vi "dfd_FXPSimu Casting (vector).vi"(7 "FXP op":T4={"source"=6, "is floating?"=FALSE, "o-mode"=enum."Wrap", "q-mode"=enum."Nearest", "signed?"=FALSE, "fwl"=0, "high limit"=0.0, "low limit"=0.0, "full range"=0.0} {"source" items=["Coef a/k"=0, "Coef b/v"=7, "Input"=1, "Output"=2, "Multiplicand"=3, "Product"=4, "Sum"=5, "Delay"=6, "Gain"=8]}, 8 "filtering statistics in":T3(array[cluster]) {"statistics information"."min value" format="%.2f"; "statistics information"."max value" format="%.2f"; "Quantizer Source" items=["Coefficients a/k"=0, "Coefficients b/v"=7, "Input"=1, "Output"=2, "Multiplicand"=3, "Product"=4, "Sum"=5, "Delay"=6]}, 11 "values in":ext[](array[numeric]) format="%.2f") -> (0 "filtering statistics out":T3(array[cluster]) {"statistics information"."min value" format="%.2f"; "statistics information"."max value" format="%.2f"; "Quantizer Source" items=["Coefficients a/k"=0, "Coefficients b/v"=7, "Input"=1, "Output"=2, "Multiplicand"=3, "Product"=4, "Sum"=5, "Delay"=6]}, 3 "values out":ext[](array[numeric]) format="%.2f")   [LabVIEW 2017, in "NI_DigFilter_FXP.lvlib"]
uses:
  <vilib>/addons/Digital Filter Design/NI_DigFilter_FXP.lvlib
  <vilib>/addons/Digital Filter Design/_Objects.llb/dfd_FXP Operation.ctl
  <vilib>/addons/Digital Filter Design/_Objects.llb/dfd_Internal Quantization Srcs.ctl
  <vilib>/addons/Digital Filter Design/_Objects.llb/DFD Quantization Sources.ctl
  <vilib>/addons/Digital Filter Design/_Objects.llb/DFD FXP Statistics Data.ctl
  <vilib>/addons/Digital Filter Design/NI_DigFilterLicensed.lvlib
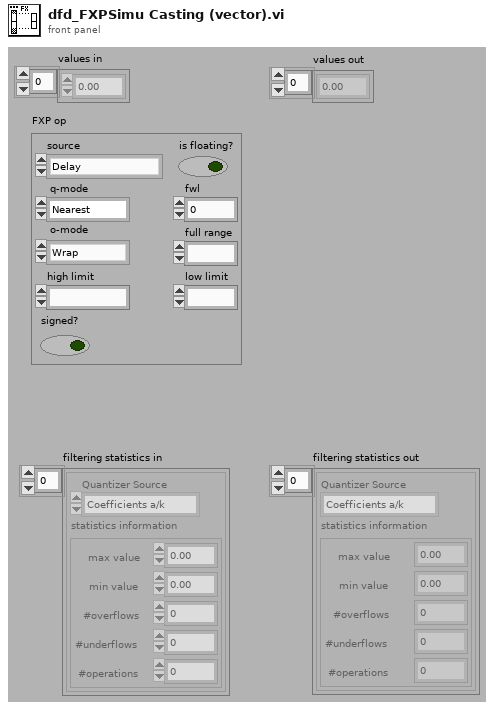
[diagram p1: front panel]
types:
  T1 = typedef "NI_DigFilterLicensed.lvlib/DFD Quantization Sources.ctl" = u16
  T2 = typedef "NI_DigFilterLicensed.lvlib/DFD FXP Statistics Data.ctl" = cluster{"max value":ext, "min value":ext, "#overflows":i32, "#underflows":i32, "#operations":i32}
  T3 = cluster{"Quantizer Source":T1, "statistics information":T2}[]
  T4 = typedef "dfd_FXP Operation.ctl" = cluster{"source":T5, "is floating?":bool, "o-mode":enum16{"Saturation", "Wrap"}, "q-mode":enum16{"Nearest", "Truncation"}, "signed?":bool, "fwl":i16, "high limit":ext, "low limit":ext, "full range":ext}
  T5 = typedef "NI_DigFilterLicensed.lvlib/dfd_Internal Quantization Srcs.ctl" = u16
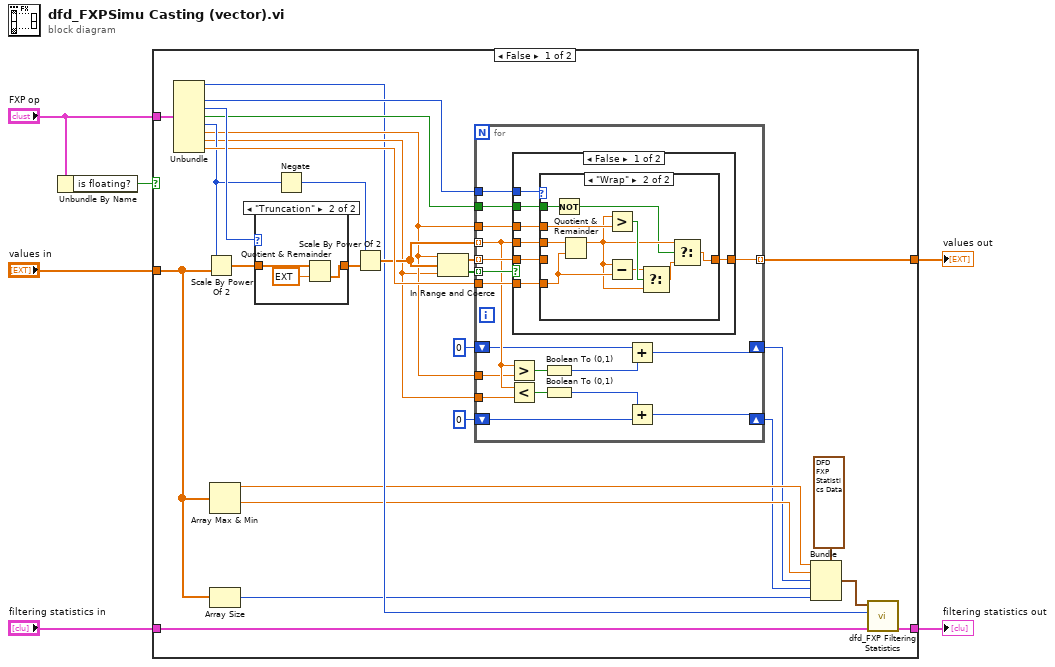
[diagram p0: block diagram]
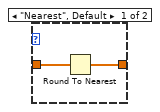
[diagram p4: hidden frame]
diagram:
  n1 = Unbundle By Name("FXP op") -> ("is floating?"=w1:bool)
  n2 = case shown="False" w1 {
    tunnel: [w34 w78] -> w6
    tunnel: "FXP op" -> [w33 _]
    tunnel: "filtering statistics in" -> [w8 w77]
    tunnel: "values in" -> [w24 w78]
    tunnel: [w7 w77] -> w2
    frame False {
      n3 = Unbundle(w33) -> ("source"=w16:T5, "o-mode"=w26:enum16{"Saturation", "Wrap"}, "q-mode"=w31:enum16{"Nearest", "Truncation"}, "signed?"=w27:bool, "fwl"=w22:i16, "high limit"=w20:ext, "low limit"=w19:ext, "full range"=w28:ext)  [unwired: 1 out]
      n4 = Scale By Power Of 2(n=w22, x=w24) -> (x*2^n=w32:ext[])
      n5 = Array Max & Min(array=w24) -> (max value=w14:ext, min value=w13:ext)  [unwired: 2 out]
      n6 = Array Size(array=w24) -> (size(s)=w10:i32)
      n7 = case shown="\"Truncation\"" w31 {
        tunnel: w32 -> [w73 w76]
        tunnel: [w72 w74] -> w25
        frame "Nearest", Default {
          n8 = Round To Nearest(number=w73) -> (nearest integer value=w72:ext[])
        }
        frame "Truncation" {
          n9 = Quotient & Remainder(x=w76, y=ext 1.0) -> (floor(x/y)=w74:ext[])  [unwired: 1 out]
        }
      }
      n10 = Negate(x=w22) -> (-x=w21:i16)
      n11 = Scale By Power Of 2(n=w21, x=w25) -> (x*2^n=w23:ext[])
      n12 = In Range and Coerce(upper limit=w20, x=w23, lower limit=w19) -> (coerced(x)=w29:ext[], In Range?=w30:bool[])
      n13 = for {
        tunnel: [w52] -> w34 mode=indexing
        tunnel: w30 -> [w51] mode=indexing
        tunnel: w29 -> [w50] mode=indexing
        tunnel: w20 -> [w49]
        tunnel: w28 -> [w48]
        tunnel: w27 -> [w47]
        tunnel: w26 -> [w46]
        tunnel: w23 -> [w45] mode=indexing
        tunnel: w20 -> [w44]
        tunnel: w19 -> [w43]
        shift-right: [w36] -> w12
        shift-left: 0 -> [w40]
        shift-right: [w35] -> w11
        shift-left: 0 -> [w38]
        n14 = Greater?(x=w45, y=w44) -> (0:w42:bool)
        n15 = Less?(x=w45, y=w43) -> (x < y?=w41:bool)
        n16 = case shown="False" w51 {
          tunnel: [w57 w71] -> w52
          tunnel: w50 -> [w58 w71]
          tunnel: w46 -> [w59 _]
          tunnel: w48 -> [w56 _]
          tunnel: w45 -> [w55 _]
          tunnel: w47 -> [w54 _]
          tunnel: w49 -> [w53 _]
          frame False {
            n17 = case shown="\"Wrap\"" w59 {
              tunnel: [w60 w69] -> w57
              tunnel: w58 -> [w60 _]
              tunnel: w56 -> [_ w64]
              tunnel: w55 -> [_ w70]
              tunnel: w54 -> [_ w68]
              tunnel: w53 -> [_ w67]
              frame "Saturation", Default {
              }
              frame "Wrap" {
                n18 = Not(x=w68) -> (.not. x?=w61:bool)
                n19 = Quotient & Remainder(x=w70, y=w64) -> (x-y*floor(x/y)=w63:ext)  [unwired: 1 out]
                n20 = Greater?(x=w63, y=w67) -> (0:w66:bool)
                n21 = Subtract(x=w63, y=w64) -> (x-y=w65:ext)
                n22 = Select(t=w65, s=w66, f=w63) -> (s? t:f=w62:ext)
                n23 = Select(t=w63, s=w61, f=w62) -> (s? t:f=w69:ext)
              }
            }
          }
          frame True {
          }
        }
        n24 = Boolean To (0,1)(Boolean=w42) -> (0, 1=w39:i16)
        n25 = Boolean To (0,1)(Boolean=w41) -> (0, 1=w37:i16)
        n26 = Add(x=w40, y=w39) -> (x+y=w36:i32)
        n27 = Add(x=w37, y=w38) -> (x+y=w35:i32)
      }
      n28 = Bundle(cluster=T2 {"max value"=-inf, "min value"=inf, "#overflows"=0, "#underflows"=0, "#operations"=1} ("new data"), "max value"=w14, "min value"=w13, "#overflows"=w12, "#underflows"=w11, "#operations"=w10) -> (w9:T2)
      n29 = call <vilib>:"dfd_FXP Filtering Statistics.vi"("filtering statistics in"=w8, "source"=w16, "new data"=w9) -> ("filtering statistics out"=w7:T3)  [unwired: 8 in]
    }
    frame True {
    }
  }
  "values out" <- w6
  "filtering statistics out" <- w2
